vi "configure operation.vi"(7 "EthernetIP configuration":refnum<class "EthernetIP configuration.lvclass">=refnum, 8 "error in":errorcluster, 10 "line item in":T1={"eip channels"=refnum, "tag name"=""}, 11 "engine configuration in":refnum<class "engine configuration.lvclass">) -> (0 "error out":errorcluster, 1 "success":bool, 2 "line item out":T1, 5 "changed":bool)   [LabVIEW 2013, in "EIP Tag API editor node.lvclass"]
uses:
  EIP Tag API editor node.lvclass
  <vilib>/NI/Module Execution Interface/Engine Configuration/engine configuration.lvclass
  <vilib>/NI/TBM Modules/Ethernet IP/channel/EthernetIP Channel.lvclass
  <vilib>/NI/Tag Bus/tag/Data Type.ctl
  <vilib>/NI/Tag Bus/tag/tag descriptor.lvclass
  <vilib>/NI/TBM Modules/Ethernet IP/configuration/EthernetIP configuration.lvclass
  table line.ctl
panel:
  in  "refresh tags":bool
  in  "Tag":i32(listbox)
  in  "Type":i32(listbox)
  in  "Instance":i32(listbox)
  out "problem":string
  in  "subindex":i32 min=0 max=7 step=1
  in  "byte index":i32
  in  "Channel Name":string
  in  "cancel":bool
  in  "ok":bool
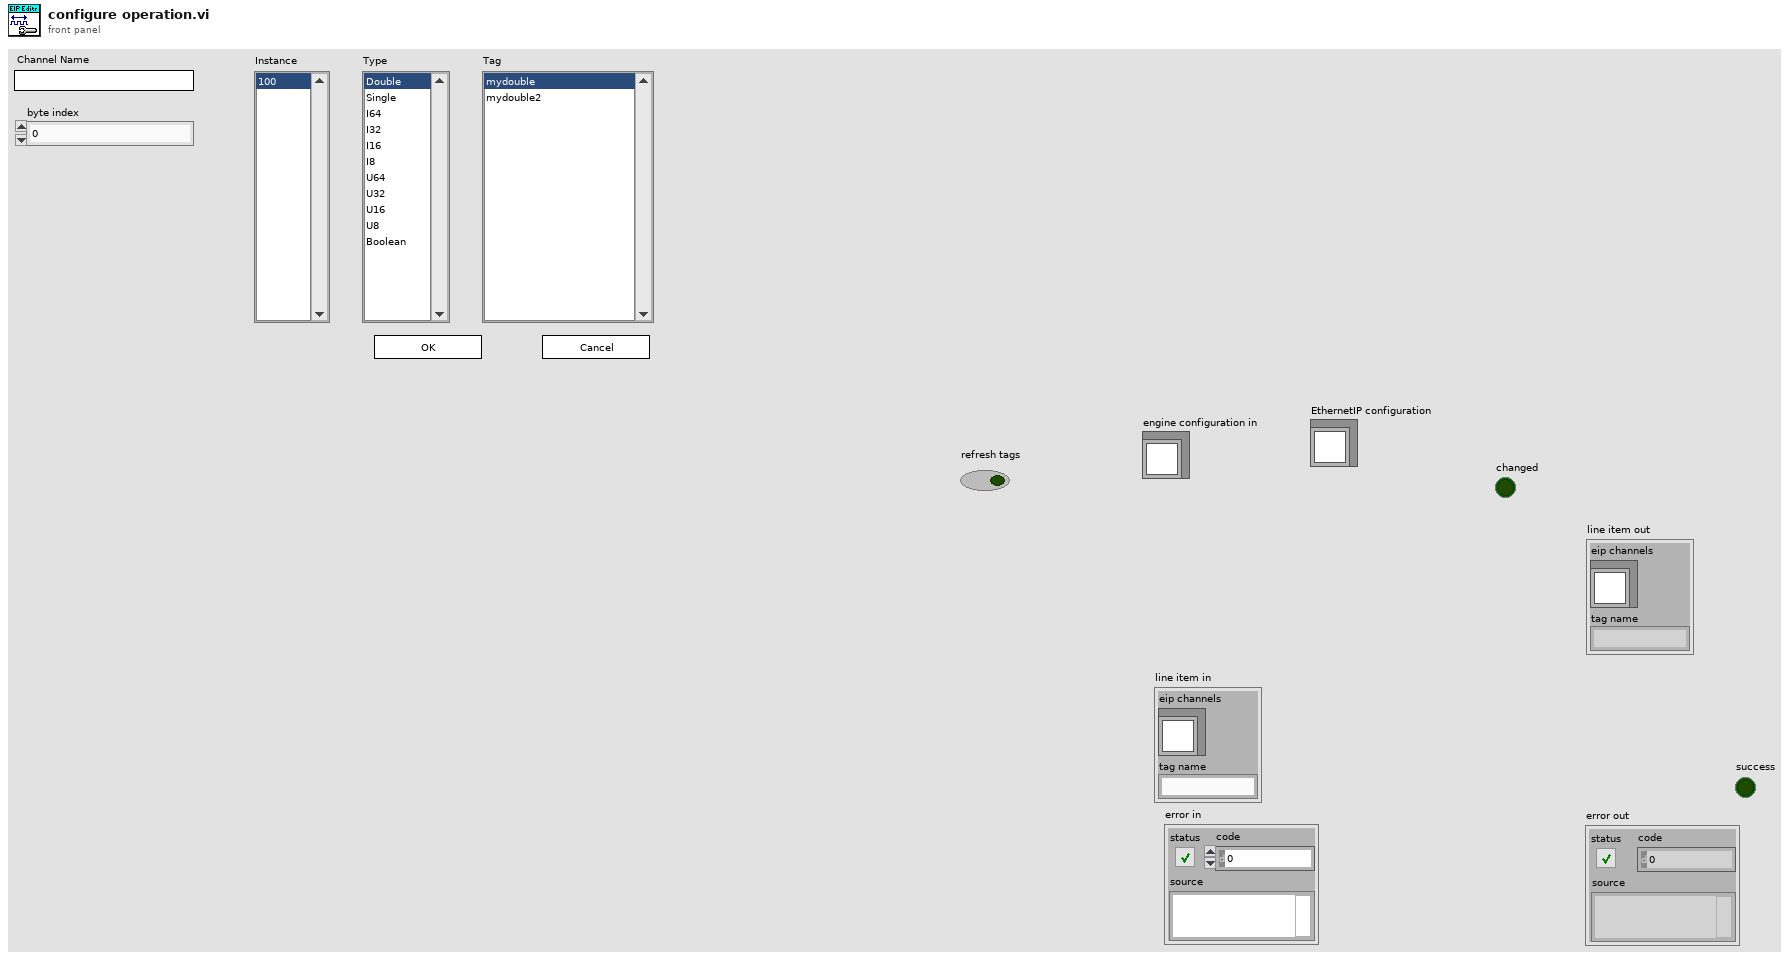
[diagram p1: front panel]
types:
  T1 = typedef "EthernetIP editor node.lvclass/table line.ctl" = cluster{"eip channels":refnum<class "EthernetIP Channel.lvclass">, "tag name":string}
  T2 = enum32{"Invalid", "Standard", "Closed", "Hidden", "Minimized", "Maximized"}
  T3 = enum32{"Invalid", "Default", "Floating", "Floating/Auto-Hide", "Modal"}
  T4 = enum8{"Enabled", "Disabled", "Disabled and Grayed Out"}
  T5 = typedef "tag bus.lvlib/tag descriptor.lvclass/Data Type.ctl" = enum16{"Double", "Single", "I64", "I32", "I16", "I8", "U64", "U32", "U16", "U8", "Boolean", "String", "Array of Double", "Array of Single", "Array of I64", "Array of I32", "Array of I16", "Array of I8", "Array of U64", "Array of U32", "Array of U16", "Array of U8", "Array of Boolean", "Array of String"}
  T6 = enum32{"invalid app kind", "Development System", "Run Time System", "Student Edition", "Embedded LabVIEW", "Evaluation", "Custom"}
  T7 = typedef "TBM channel.lvclass/channel classification.ctl" = enum16{"input data", "output data", "processing parameter", "processing result"}
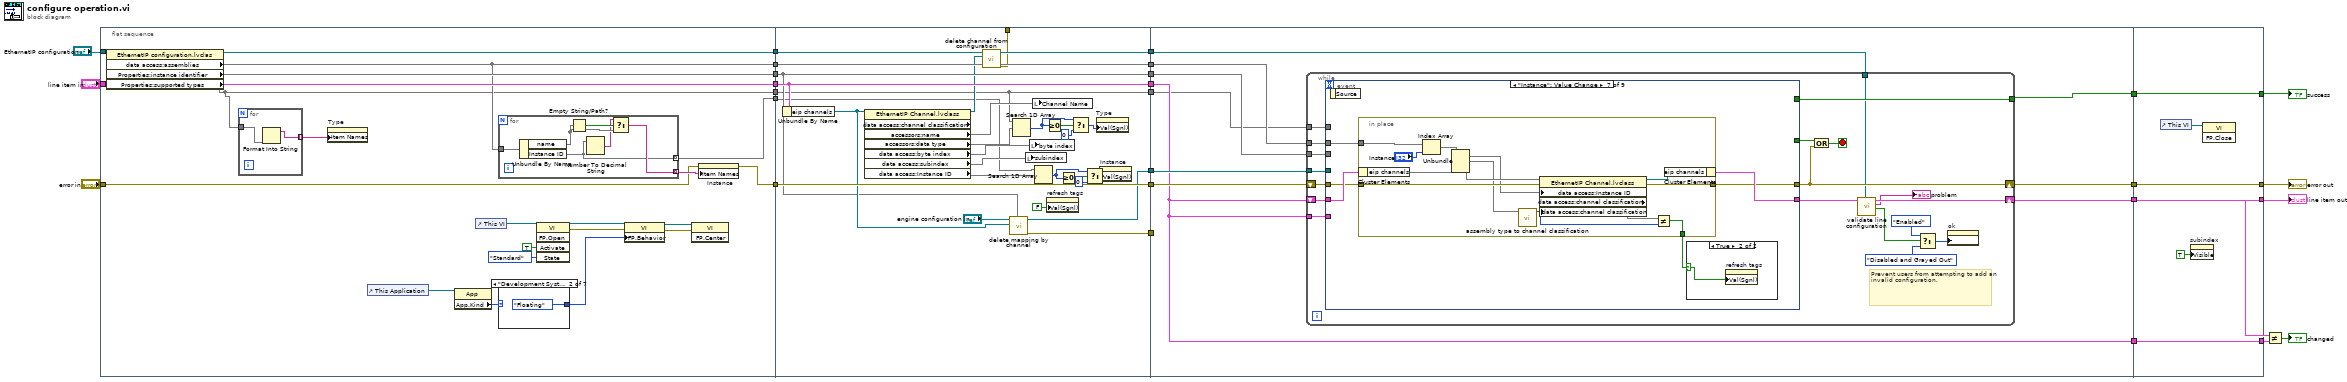
[diagram p0: block diagram]
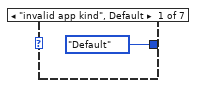
[diagram p2: hidden frame]
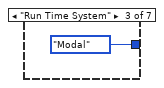
[diagram p3: hidden frame]
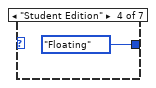
[diagram p4: hidden frame]
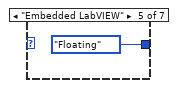
[diagram p5: hidden frame]
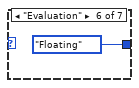
[diagram p6: hidden frame]
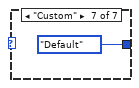
[diagram p7: hidden frame]
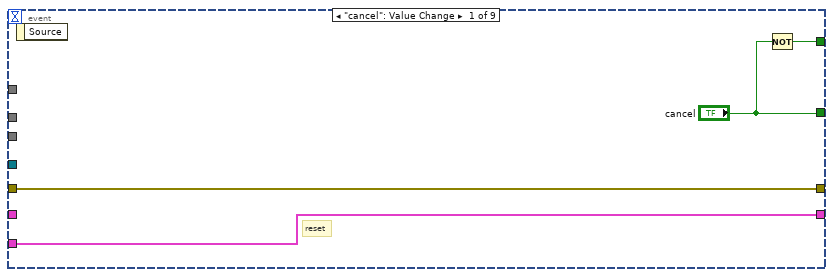
[diagram p8: hidden frame]
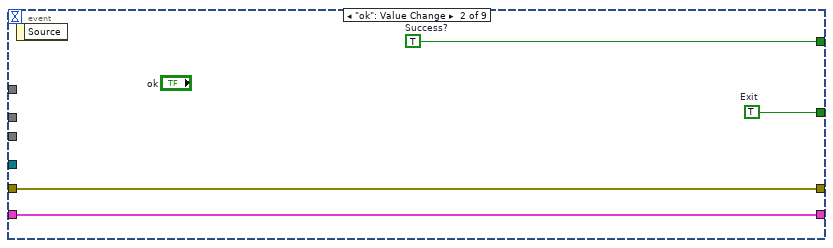
[diagram p9: hidden frame]
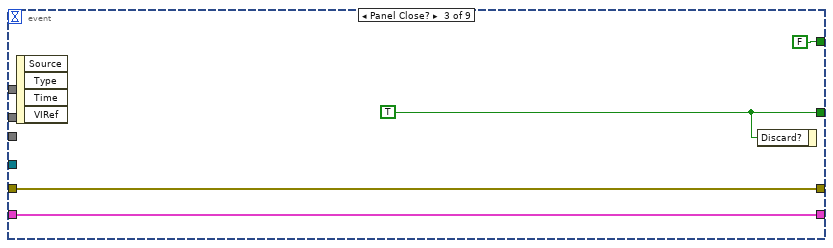
[diagram p10: hidden frame]
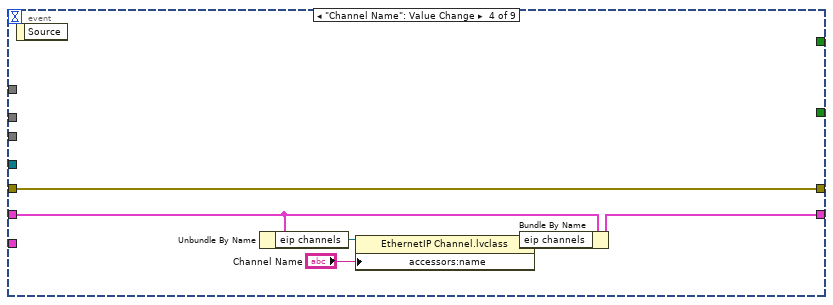
[diagram p11: hidden frame]
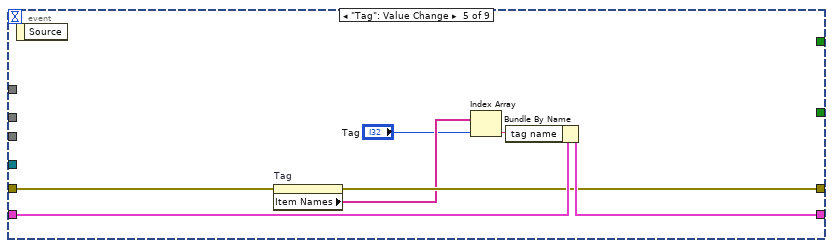
[diagram p12: hidden frame]
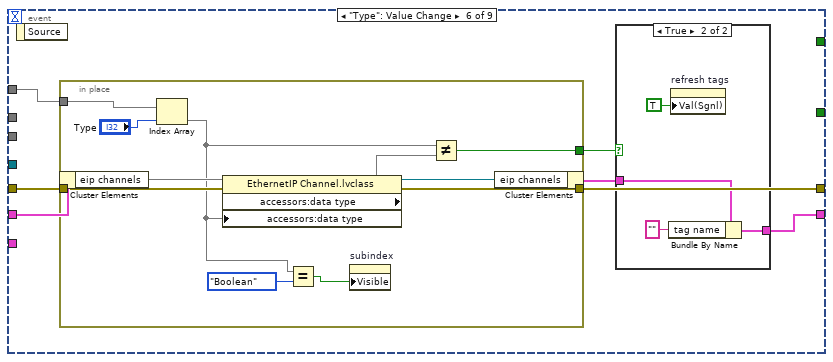
[diagram p13: hidden frame]
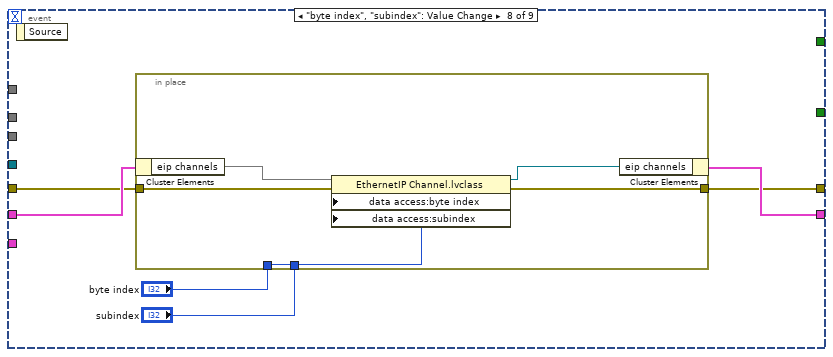
[diagram p16: hidden frame]
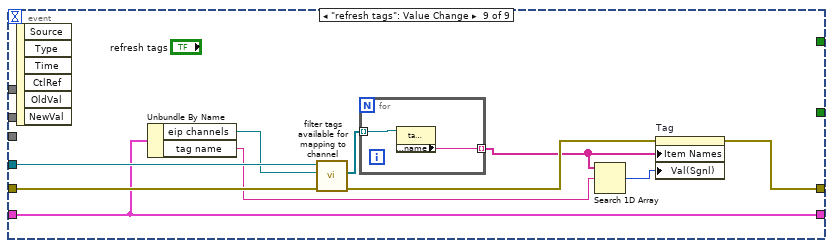
[diagram p17: hidden frame]
diagram:
  n1 = flat-sequence {
    tunnel: "line item in" -> [w48]
    tunnel: "error in" -> [w34]
    tunnel: [w33] -> w16
    tunnel: [w48] -> w14
    tunnel: "EthernetIP configuration" -> [w39]
    tunnel: [w38] -> w8
    tunnel: [w36] -> w6
    tunnel: [w37] -> w5
    tunnel: [w32] -> w2
    tunnel: [w30] -> w1
    tunnel: w16 -> [w91]
    tunnel: [w91] -> w15
    tunnel: w14 -> [w89]
    tunnel: [w89] -> w13
    tunnel: [w87] -> w12
    tunnel: [w86] -> w11
    tunnel: [w79] -> w9
    tunnel: w8 -> [w82]
    tunnel: [w81] -> w7
    tunnel: w6 -> [w81]
    tunnel: w5 -> [w80]
    tunnel: [w80] -> w4
    tunnel: [w77] -> _
    tunnel: [w76] -> w3
    tunnel: w2 -> [w76]
    tunnel: w1 -> [w70]
    tunnel: [w100] -> w20
    tunnel: [w99] -> w19
    tunnel: [w98] -> w18
    tunnel: [w93] -> w17
    tunnel: w15 -> [w101]
    tunnel: w13 -> [w93]
    tunnel: w12 -> [_]
    tunnel: w11 -> [w97]
    tunnel: w9 -> [w96]
    tunnel: w7 -> [w95]
    tunnel: w4 -> [w94]
    tunnel: w3 -> [w92]
    tunnel: [w213] -> w21
    tunnel: [w214] -> w24
    tunnel: [w215] -> w25
    tunnel: [w216] -> w26
    tunnel: w20 -> [w216]
    tunnel: w19 -> [w215]
    tunnel: w18 -> [w214]
    tunnel: w17 -> [w213]
    frame #0 {
      n2 = property class="EthernetIP configuration.lvclas"(reference=w39) -> (reference out=w38:refnum<class "EthernetIP configuration.lvclass">, "data access:assemblies"=w36, "Properties:instance identifier"=w37, "Properties:supported types"=w32)  [unwired: 1 in, 1 out]
      n3 = for {
        tunnel: w32 -> [w50]
        tunnel: [w49] -> w31 mode=indexing
        n4 = Format Into String(w50) -> (resulting string=w49:string)  [unwired: 3 in, 1 out]
      }
      n5 = property on="Type" class="LstBox (strict)"("Item Names"=w31) -> ()  [unwired: 2 in, 2 out]
      n6 = control-ref of="This Application"() -> (w42:refnum<vi>)
      n7 = property class="App"(reference=w42) -> ("App.Kind"=w41:T6)  [unwired: 1 in, 2 out]
      n8 = control-ref of="This VI"() -> (w43:refnum<vi>)
      n9 = for {
        tunnel: w36 -> [w56]
        tunnel: [w52] -> w35 mode=indexing
        tunnel: [w51] -> w30 mode=indexing
        n10 = Unbundle By Name(w56) -> ("name"=w54, "Instance ID"=w51)
        n11 = Empty String/Path?(string/path=w54) -> (empty?=w55:bool)
        n12 = Number To Decimal String(number=w51) -> (decimal integer string=w53:string)  [unwired: 1 in]
        n13 = Select(t=w53, s=w55, f=w54) -> (s? t:f=w52:string)
      }
      n14 = case shown="\"Development System\"" w41 {
        tunnel: [T3."Default" ("Front Panel Window:Behavior") T3."Floating" ("Front Panel Window:Behavior") T3."Modal" ("Front Panel Window:Behavior") T3."Floating" ("Front Panel Window:Behavior") T3."Floating" ("Front Panel Window:Behavior") T3."Floating" ("Front Panel Window:Behavior") T3."Default" ("Front Panel Window:Behavior")] -> w40
        frame "invalid app kind", Default {
        }
        frame "Development System" {
        }
        frame "Run Time System" {
        }
        frame "Student Edition" {
        }
        frame "Embedded LabVIEW" {
        }
        frame "Evaluation" {
        }
        frame "Custom" {
        }
      }
      n15 = invoke class="VI" method="FP.Open"(reference=w43, "Activate"=TRUE ("Activate?"), "State"=T2."Standard") -> (reference out=w46:refnum<vi>, error out=w47:errorcluster)  [unwired: 2 in, 3 out]
      n16 = property class="VI"(reference=w46, error in=w47, "FP.Behavior"=w40) -> (reference out=w29:refnum<vi>, error out=w28:errorcluster)
      n17 = invoke class="VI" method="FP.Center"(reference=w29, error in=w28) -> ()  [unwired: 1 in, 3 out]
      n18 = property on="Instance" class="LstBox (strict)"(error in=w34, "Item Names"=w35) -> (error out=w33:errorcluster)  [unwired: 1 in, 1 out]
    }
    frame #1 {
      n19 = Unbundle By Name(w89) -> ("eip channels"=w85:refnum<class "EthernetIP Channel.lvclass">)
      n20 = property class="EthernetIP Channel.lvclass" props=["data access:channel classification", "accessors:name", "accessors:data type", "data access:byte index", "data access:subindex", "data access:Instance ID"](reference=w85) -> (reference out=w78:refnum<class "EthernetIP Channel.lvclass">, "accessors:name"=w90, "accessors:data type"=w75, "data access:byte index"=w84, "data access:subindex"=w83, "data access:Instance ID"=w65)  [unwired: 1 in, 2 out]
      n21 = call <vilib>:"delete channel from configuration.vi"("TBM channel in"=w78, "EthernetIP configuration in"=w82) -> ("error out"=w77:errorcluster, "EthernetIP configuration out"=w79:refnum<class "EthernetIP configuration.lvclass">)  [unwired: 8 in]
      n22 = call <vilib>:"delete mapping by channel.vi"("owner ID"=w80, "channel"=w85, "engine configuration in"="engine configuration in") -> ("error out"=w87:errorcluster, "engine configuration out"=w86:refnum<class "engine configuration.lvclass">)  [unwired: 7 in]
      n23 = Search 1D Array(1D array=w76, element=w75) -> (index of element=w73:i32)  [unwired: 1 in]
      n24 = local write "subindex"(w83) -> ()
      n25 = local write "byte index"(w84) -> ()
      n26 = local write "Channel Name"(w90) -> ()
      n27 = Search 1D Array(1D array=w70, element=w65) -> (index of element=w67:i32)  [unwired: 1 in]
      n28 = Greater Or Equal To 0?(x=w73) -> (x >= 0?=w74:bool)
      n29 = property on="refresh tags" class="Bool (strict)"("Val(Sgnl)"=FALSE ("Value (Signaling)")) -> ()  [unwired: 2 in, 2 out]
      n30 = Greater Or Equal To 0?(x=w67) -> (x >= 0?=w68:bool)
      n31 = Select(t=w73, s=w74, f=0) -> (s? t:f=w71:i32)
      n32 = Select(t=w67, s=w68, f=0) -> (s? t:f=w66:i32)
      n33 = property on="Type" class="LstBox (strict)"("Val(Sgnl)"=w71) -> ()  [unwired: 2 in, 2 out]
      n34 = property on="Instance" class="LstBox (strict)"("Val(Sgnl)"=w66) -> ()  [unwired: 2 in, 2 out]
    }
    frame #2 {
      n35 = while {
        shift-right: [w111] -> w99
        shift-left: w101 -> [w119]
        tunnel: [w118] -> w100
        shift-right: [w112] -> w98
        shift-left: w93 -> [w115]
        tunnel: w93 -> [w114]
        tunnel: w97 -> [w120]
        tunnel: w96 -> [w106]
        tunnel: w95 -> [w105]
        tunnel: w94 -> [w104]
        tunnel: w92 -> [w102]
        stop <- w116 stop-if-true
        # "Prevent users from attempting to add an invalid configuration."
        n36 = event shown="[6] \"Instance\": Value Change" {
          selector: _ -> [_ _ _ _ _ _ _ _ _]
          dyn-events: _ -> [_ _ _ _ _ _ _ _ _]
          timeout: _ -> [_ _ _ _ _ _ _ _ _]
          tunnel: w120 -> [_ _ _ _ _ _ _ _ w206]
          tunnel: w119 -> [w124 w128 w132 w138 w144 w151 w172 w191 w208]
          tunnel: [w124 w128 w132 w138 w141 w150 w171 w190 w207] -> w111
          tunnel: [w123 w125 FALSE _ _ _ _ _ _] -> w118
          tunnel: ["cancel" w126 w130 _ _ _ _ _ _] -> w117
          tunnel: w115 -> [_ w127 w129 w136 w145 w152 w174 w193 w205]
          tunnel: [w121 w127 w129 w137 w143 w147 w173 w192 w205] -> w113
          tunnel: w114 -> [w121 _ _ _ _ _ _ _ _]
          tunnel: w105 -> [_ _ _ _ _ _ w169 _ _]
          tunnel: w104 -> [_ _ _ _ _ _ _ _ _]
          tunnel: w102 -> [_ _ _ _ _ w146 _ _ _]
          event "cancel": Value Change {
            # "reset"
            n37 = event-data() -> ()  [unwired: 1 in, 1 out]
            n38 = Not(x="cancel") -> (.not. x?=w123:bool)
          }
          event "ok": Value Change {
            w125 = TRUE  # Success?
            w126 = TRUE  # Exit
            n39 = event-data() -> ()  [unwired: 1 in, 1 out]
          }
          event Panel Close? {
            w130 = TRUE ("cancel")
            n40 = event-data() -> ()  [unwired: 1 in, 4 out]
            n41 = event-data("Discard?"=w130) -> ()  [unwired: 1 in, 1 out]
          }
          event "Channel Name": Value Change {
            n42 = event-data() -> ()  [unwired: 1 in, 1 out]
            n43 = Unbundle By Name(w136) -> ("eip channels"=w135:refnum<class "EthernetIP Channel.lvclass">)
            n44 = property class="EthernetIP Channel.lvclass"(reference=w135, "accessors:name"="Channel Name") -> (reference out=w134:refnum<class "EthernetIP Channel.lvclass">)  [unwired: 1 in, 1 out]
            n45 = Bundle By Name(cluster=w136, "eip channels"=w134) -> (w137:T1)
          }
          event "Tag": Value Change {
            n46 = event-data() -> ()  [unwired: 1 in, 1 out]
            n47 = property on="Tag" class="LstBox (strict)"(error in=w144) -> (error out=w141:errorcluster, "Item Names"=w140:string[])  [unwired: 1 in, 1 out]
            n48 = Index Array(array=w140, index="Tag") -> (element=w142:string)
            n49 = Bundle By Name(cluster=w145, "tag name"=w142) -> (w143:T1)
          }
          event "Type": Value Change {
            n50 = event-data() -> ()  [unwired: 1 in, 1 out]
            n51 = in-place {
              in-place-border: w151 -> [w167]
              in-place-border: [w166] -> w150
              in-place-border: [w161] -> w149
              in-place-border: w146 -> [w160]
              n52 = in-place-cluster #1(w152) -> ("eip channels"=w168)
              n53 = Index Array(array=w160, index="Type") -> (element=w158)
              n54 = property class="EthernetIP Channel.lvclass"(reference=w168, error in=w167, "accessors:data type"=w158) -> (reference out=w165:refnum<class "EthernetIP Channel.lvclass">, error out=w166:errorcluster, "accessors:data type"=w162)
              n55 = Equal?(x=w158, y=Data_Type."Boolean") -> (x = y?=w163:bool)
              n56 = property on="subindex" class="DigNum (strict)"("Visible"=w163) -> ()  [unwired: 2 in, 2 out]
              n57 = Not Equal?(x=w158, y=w162) -> (x != y?=w161:bool)
              n58 = in-place-cluster #1("eip channels"=w165) -> (w148:cluster{})
            }
            n59 = case shown="True" w149 {
              tunnel: w148 -> [w153 w156]
              tunnel: [w153 w155] -> w147
              frame False {
              }
              frame True {
                n60 = Bundle By Name(cluster=w156, "tag name"="") -> (w155:cluster{})
                n61 = property on="refresh tags" class="Bool (strict)"("Val(Sgnl)"=TRUE ("Value (Signaling)")) -> ()  [unwired: 2 in, 2 out]
              }
            }
          }
          event "Instance": Value Change {
            n62 = event-data() -> ()  [unwired: 1 in, 1 out]
            n63 = in-place {
              in-place-border: w172 -> [w187]
              in-place-border: [w186] -> w171
              in-place-border: [w181] -> w170
              in-place-border: w169 -> [w179]
              n64 = in-place-cluster #2(w174) -> ("eip channels"=w185)
              n65 = Index Array(array=w179, index="Instance") -> (element=w178)
              n66 = Unbundle(w178) -> (w177, w176)  [unwired: 3 out]
              n67 = call <vilib>:"assembly type to channel classification.vi"("Type"=w176) -> ("channel classification"=w182:T7)  [unwired: 10 in]
              n68 = property class="EthernetIP Channel.lvclass"(reference=w185, error in=w187, "data access:Instance ID"=w177, "data access:channel classification"=w182) -> (reference out=w184:refnum<class "EthernetIP Channel.lvclass">, error out=w186:errorcluster, "data access:channel classification"=w183)
              n69 = Not Equal?(x=w183, y=w182) -> (x != y?=w181:bool)
              n70 = in-place-cluster #2("eip channels"=w184) -> (w173:cluster{})
            }
            n71 = case shown="True" w170 {
              selector: w170 -> [_ w175]
              frame False {
              }
              frame True {
                n72 = property on="refresh tags" class="Bool (strict)"("Val(Sgnl)"=w175) -> ()  [unwired: 2 in, 2 out]
              }
            }
          }
          event "byte index", "subindex": Value Change {
            n73 = event-data() -> ()  [unwired: 1 in, 1 out]
            n74 = in-place {
              in-place-border: w191 -> [w199]
              in-place-border: [w198] -> w190
              in-place-border: "subindex" -> [w195]
              in-place-border: "byte index" -> [w194]
              n75 = in-place-cluster #3(w193) -> ("eip channels"=w197)
              n76 = property class="EthernetIP Channel.lvclass"(reference=w197, error in=w199, "data access:byte index"=w194, "data access:subindex"=w195) -> (reference out=w196:refnum<class "EthernetIP Channel.lvclass">, error out=w198:errorcluster)
              n77 = in-place-cluster #3("eip channels"=w196) -> (w192:cluster{})
            }
          }
          event "refresh tags": Value Change {
            n78 = event-data() -> ()  [unwired: 1 in, 6 out]
            n79 = Unbundle By Name(w205) -> ("eip channels"=w204:refnum<class "EthernetIP Channel.lvclass">, "tag name"=w201:string)
            n80 = call <vilib>:"filter tags available for mapping to channel.vi"("channel to map to"=w204, "engine configuration in"=w206) -> ("filtered tags"=w203:refnum<class "tag descriptor.lvclass">[])  [unwired: 8 in, 1 out]
            n81 = for {
              tunnel: w203 -> [w210] mode=indexing
              tunnel: [w209] -> w202 mode=indexing
              n82 = property class="tag descriptor"(reference=w210) -> ("accessors:name"=w209:string)  [unwired: 1 in, 2 out]
            }
            n83 = Search 1D Array(1D array=w202, element=w201) -> (index of element=w200:i32)  [unwired: 1 in]
            n84 = property on="Tag" class="LstBox (strict)"(error in=w208, "Item Names"=w202, "Val(Sgnl)"=w200) -> (error out=w207:errorcluster)  [unwired: 1 in, 1 out]
          }
        }
        n85 = Compound Arithmetic op=OR(w117, w111) -> (w116:bool)
        n86 = call "validate line configuration.vi"("EthernetIP configuration"=w106, "line in"=w113) -> ("valid?"=w110:bool, "problem"=→"problem":string, "line out"=w112:T1)  [unwired: 7 in]
        n87 = Select(t=T4."Enabled" ("Disabled"), s=w110, f=T4."Disabled and Grayed Out") -> (s? t:f=w107:T4)
        n88 = property on="ok" class="Bool"("DisabledEnum"=w107) -> ()  [unwired: 2 in, 2 out]
      }
    }
    frame #3 {
      n89 = control-ref of="This VI"() -> (w212:refnum<vi>)
      n90 = property on="subindex" class="DigNum (strict)"("Visible"=TRUE) -> ()  [unwired: 2 in, 2 out]
      n91 = invoke class="VI" method="FP.Close"(reference=w212) -> ()  [unwired: 2 in, 3 out]
    }
  }
  n92 = Not Equal?(x=w24, y=w21) -> (x != y?=→"changed":bool)
  "error out" <- w25
  "success" <- w26
  "line item out" <- w24
